vi "Progressbar_Create.vi"(7 "Object Attributes":T2, 8 "error in (no error)":errorcluster, 9 "Progressbar Attributes":T1, 10 "Control Attributes":T4, 11 "Progress In":refnum<class "Progressbar.lvclass">) -> (0 "error out":errorcluster, 3 "Progress Out":refnum<class "Progressbar.lvclass">)   [LabVIEW 2015, in "Front Panel Publisher.lvlib" / "Progressbar.lvclass"]
uses:
  Progressbar.lvclass
  Control_class/Control.lvclass
  Attributes.ctl
  Object_class/Coordinates.ctl
  Object_class/Object.lvclass
  Object_class/Attributes.ctl
  Text_class/Text.lvclass
  Control_class/Attributes.ctl
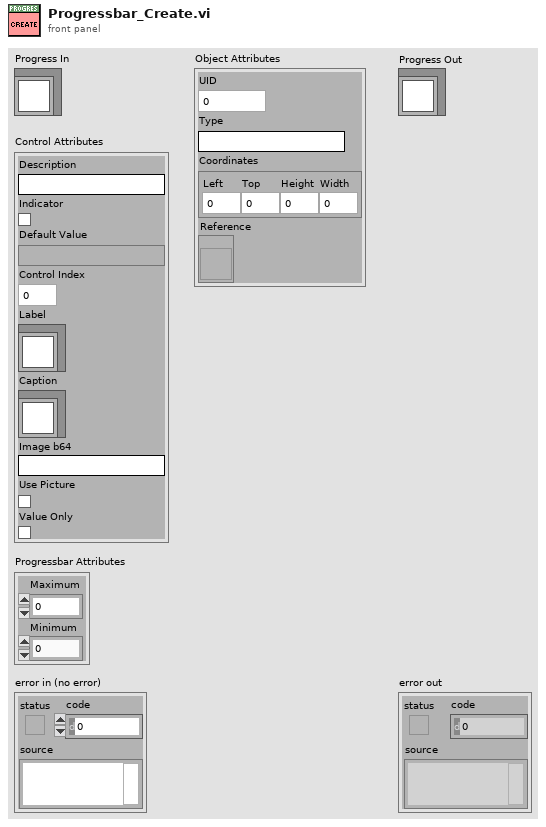
[diagram p1: front panel]
types:
  T1 = typedef "Front Panel Publisher.lvlib/Progressbar.lvclass/Attributes.ctl" = cluster{"Maximum":dbl, "Minimum":dbl}
  T2 = typedef "Front Panel Publisher.lvlib/Object.lvclass/Attributes.ctl" = cluster{"UID":i32, "Type":string, "Coordinates":T3, "Reference":refnum<vi>}
  T3 = typedef "Front Panel Publisher.lvlib/Object.lvclass/Coordinates.ctl" = cluster{"Left":i32, "Top":i32, "Height":u32, "Width":u32}
  T4 = typedef "Front Panel Publisher.lvlib/Control.lvclass/Attributes.ctl" = cluster{"Description":string, "Indicator":bool, "Default Value":variant, "Control Index":i32, "Label":refnum<class "Text.lvclass">, "Caption":refnum<class "Text.lvclass">, "Image b64":string, "Use Picture":bool, "Value Only":bool}
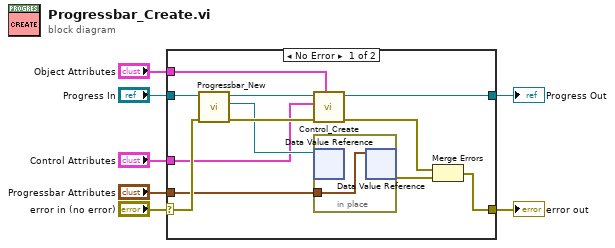
[diagram p0: block diagram]
diagram:
  n1 = case shown="No Error" "error in (no error)" {
    selector: "error in (no error)" -> [w18 w22]
    tunnel: [w16 w22] -> w6
    tunnel: "Progress In" -> [w19 w21]
    tunnel: [w13 w21] -> w4
    tunnel: "Object Attributes" -> [w11 _]
    tunnel: "Control Attributes" -> [w9 _]
    tunnel: "Progressbar Attributes" -> [w8 _]
    frame No Error {
      n2 = call "Progressbar_New.vi"("error in (no error)"=w18, "reference in"=w19) -> ("error out"=w14:errorcluster, "DVRRefOut"=w12:refnum<data-value>, "reference out"=w15:refnum<class "Progressbar.lvclass">)  [unwired: 6 in, 1 out]
      n3 = call "Control_Create.vi"("Object Attributes"=w11, "error in (no error)"=w14, "Control Attributes"=w9, "Control In"=w15) -> ("error out"=w10:errorcluster, "Control Out"=w13:refnum<class "Progressbar.lvclass">)  [unwired: 6 in]
      n4 = in-place {
        in-place-border: w8 -> [w20]
        n5 = in-place-dvr #1(w12) -> ()  [unwired: 2 out]
        n6 = in-place-dvr #1(w20) -> (w17:errorcluster)  [unwired: 1 out]
      }
      n7 = Merge Errors(w10, w17) -> (w16:errorcluster)
    }
    frame Error {
    }
  }
  "error out" <- w6
  "Progress Out" <- w4
